vi "Untitled 3.vi"() -> ()   [LabVIEW 2019]
panel:
  in  "Direction":dbl
  out "Difference":dbl
  in  "Target Position":dbl
  in  "stop":bool
  out "backRight":dbl
  out "backLeft":dbl
  out "frontRight":dbl
  out "frontLeft":dbl
  in  "gyroscope position":dbl
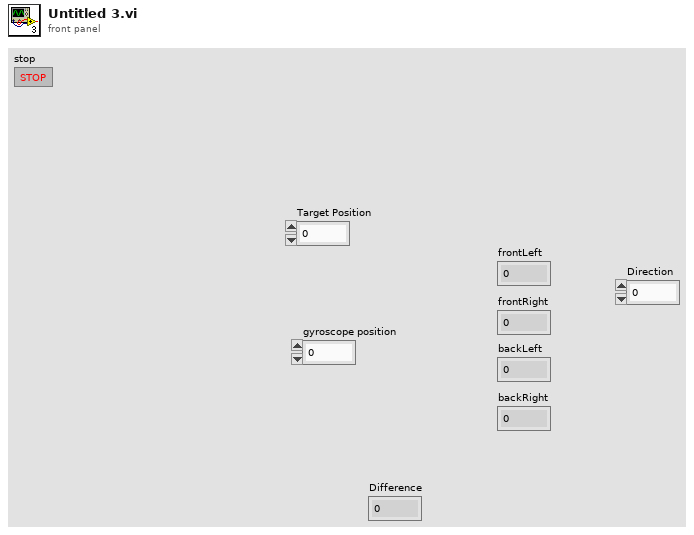
[diagram p1: front panel]
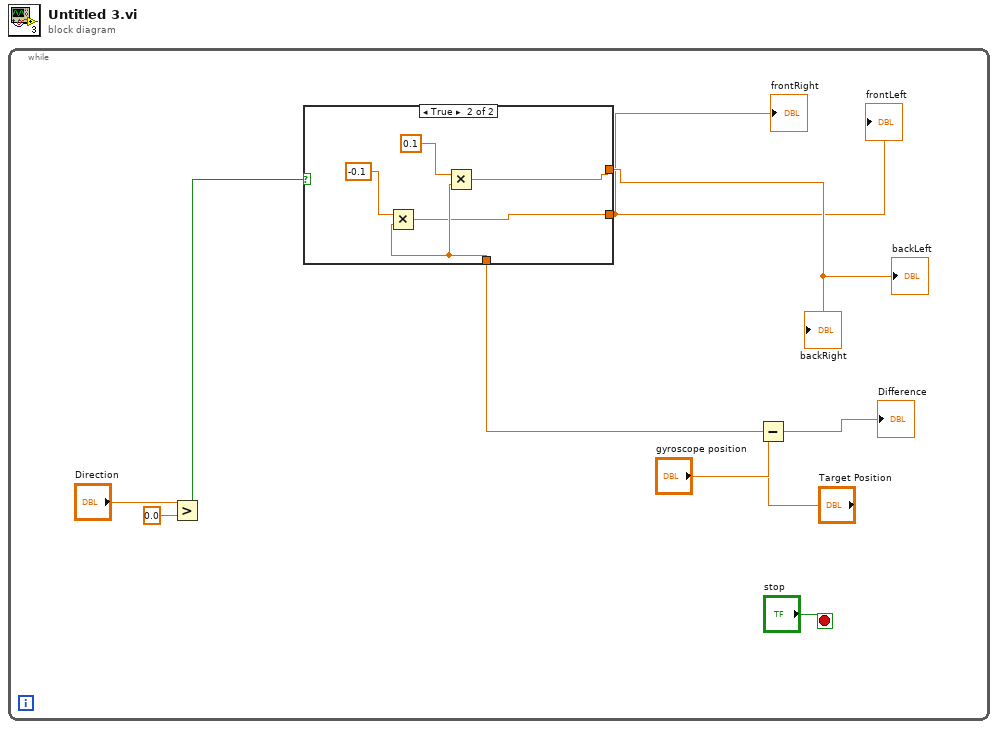
[diagram p0: block diagram]
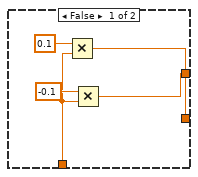
[diagram p2: hidden frame]
diagram:
  n1 = while {
    stop <- "stop" stop-if-true
    n2 = Greater?(x="Direction", y=0.0) -> (0:w4:bool)
    n3 = Subtract(x="gyroscope position", y="Target Position") -> (x-y=w3:dbl)
    "Difference" <- w3
    n4 = case shown="True" w4 {
      tunnel: w3 -> [w12 w17]
      tunnel: [w11 w16] -> w2
      tunnel: [w10 w15] -> w1
      frame False {
        n5 = Multiply(x=0.1, y=w12) -> (x*y=w10:dbl)
        n6 = Multiply(x=-0.1, y=w12) -> (x*y=w11:dbl)
      }
      frame True {
        n7 = Multiply(x=-0.1, y=w17) -> (x*y=w15:dbl)
        n8 = Multiply(x=0.1, y=w17) -> (x*y=w16:dbl)
      }
    }
    "frontLeft" <- w1
    "frontRight" <- w1
    "backLeft" <- w2
    "backRight" <- w2
  }
